vi "Stock Designs.vi"(6 "Method cmd":T1=enum."Run", 8 "error in (no error)":errorcluster, 10 "Revision":i32, 11 "Methods ring":refnum<vi>) -> (0 "error out":errorcluster, 3 "Method":T2)   [LabVIEW 2011]
uses:
  Design Server.lvlib
  Method.ctl
  Load method ring.ctl
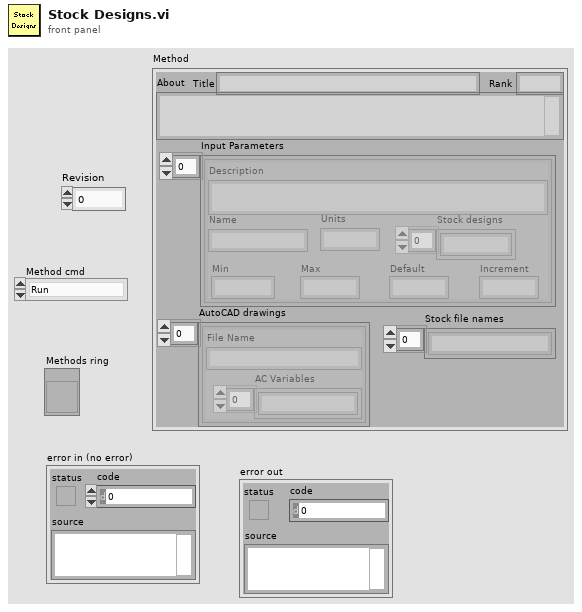
[diagram p1: front panel]
types:
  T1 = typedef "Load method ring.ctl" = enum16{"Load Method Ring", "Run"}
  T2 = typedef "Method.ctl" = cluster{"Title":string, "Rank":string, "About":string, "Input Parameters":cluster{"Description":string, "Name":string, "Min":string, "Max":string, "Default":string, "Units":string, "Increment":string, "Stock designs":string[]}[], "AutoCAD drawings":cluster{"File Name":string, "AC Variables":string[]}[], "Stock file names":string[]}
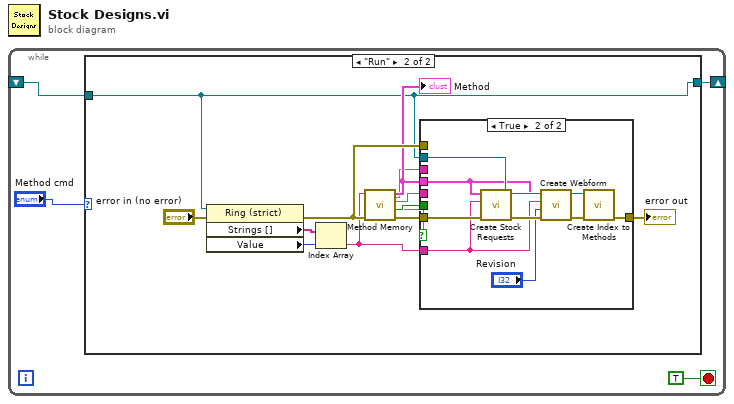
[diagram p0: block diagram]
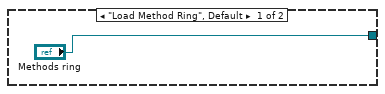
[diagram p2: hidden frame]
diagram:
  n1 = while {
    shift-right: [w3] -> _
    shift-left: _ -> [w2]
    stop <- TRUE stop-if-true
    n2 = case shown="\"Run\"" "Method cmd" {
      tunnel: w2 -> [_ w6]
      tunnel: ["Methods ring" w6] -> w3
      frame "Load Method Ring", Default {
      }
      frame "Run" {
        n3 = property class="Ring (strict)"(reference=w6, error in="error in (no error)") -> (error out=w11:errorcluster, "Strings []"=w17:string[], "Value"=w16:u16)  [unwired: 1 out]
        n4 = Index Array(array=w17, index=w16) -> (element=w8:string)
        n5 = call "Method Memory.vi"("error in"=w11, "Method Name"=w8) -> ("error out"=w14:errorcluster, "method exists?"=w12:bool, 2:w13, "Method Out"=w10:T2, 4:w9, 7:w7)  [unwired: 4 in]
        "Method" <- w10
        n6 = case shown="True" w9 {
          tunnel: [w19 w20] -> w18
          tunnel: w14 -> [w19 w27]
          tunnel: w13 -> [_ _]
          tunnel: w12 -> [_ _]
          tunnel: w11 -> [_ _]
          tunnel: w10 -> [_ w22]
          tunnel: w6 -> [_ w24]
          tunnel: w8 -> [_ w23]
          tunnel: w7 -> [_ _]
          frame False {
          }
          frame True {
            n7 = call "Create Stock Requests.vi"("error in"=w27, "Method Name"=w23, "Method"=w22) -> ("error out"=w26:errorcluster)  [unwired: 8 in]
            n8 = call "Create Webform.vi"("error in (no error)"=w26, "Revision"="Revision", "Method Name"=w23, "Method"=w22) -> ("error out"=w25:errorcluster)  [unwired: 6 in, 1 out]
            n9 = call "Create Index to Methods.vi"("error in"=w25, "Method Names"=w24) -> ("error out"=w20:errorcluster)  [unwired: 9 in]
          }
        }
        "error out" <- w18
      }
    }
  }
